vi "Exclude Test Methods from Set of VIs in Project.vi"(11 "VIs":set{path}(c389)) -> (3 "VIs 2":set{path}(c389))   [LabVIEW 2020, in "LUnit Tests.lvlib" / "Coverage Test.lvclass"]
uses:
  Coverage Test.lvclass
  Coverage Test.lvclass/Coverage Test.ctl
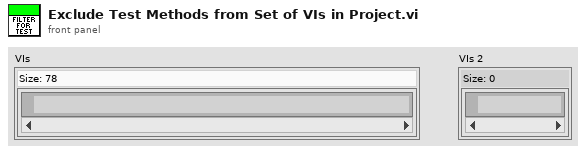
[diagram p1: front panel]
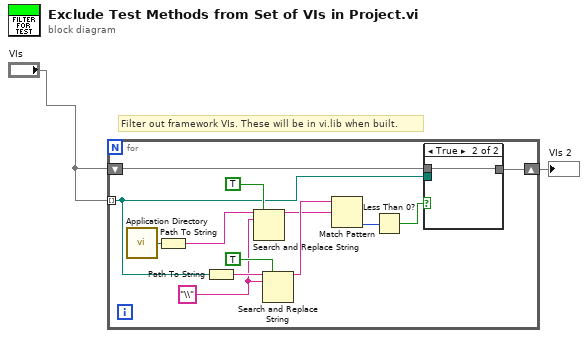
[diagram p0: block diagram]
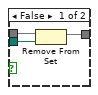
[diagram p2: hidden frame]
diagram:
  # "Filter out framework VIs. These will be in vi.lib when built."
  n1 = for {
    tunnel: "VIs" -> [w4] mode=indexing
    shift-right: [w5] -> w1
    shift-left: "VIs" -> [w6]
    w7 = "\\" ("search string")
    n2 = call <vilib>:"Application Directory.vi"() -> ("Application Directory"=w14:path)
    n3 = Path To String(path=w14) -> (string=w9:string)
    n4 = Path To String(path=w4) -> (string=w15:string)
    n5 = Search and Replace String(replace all?=TRUE ("replace all? (F)"), input string=w9, search string=w7) -> (result string=w8:string)  [unwired: 5 in, 3 out]
    n6 = Search and Replace String(replace all?=TRUE ("replace all? (F)"), input string=w15, search string=w7) -> (result string=w12:string)  [unwired: 5 in, 3 out]
    n7 = Match Pattern(string=w12, regular expression=w8) -> (offset past match=w13:i32)  [unwired: 1 in, 3 out]
    n8 = Less Than 0?(x=w13) -> (x < 0?=w3:bool)
    n9 = case shown="True" w3 {
      tunnel: w6 -> [w18 w19]
      tunnel: [w17 w19] -> w5
      tunnel: w4 -> [w16 _]
      frame False {
        n10 = Remove From Set(10:w16, 11:w18) -> (3:w17:set{path})  [unwired: 1 out]
      }
      frame True {
      }
    }
  }
  "VIs 2" <- w1
